vi "ReadDough.vi"(8 "error in (no error)":errorcluster, 11 "object in":refnum<class "Pizza.lvclass">) -> (0 "error out":errorcluster, 2 "dough":string, 3 "object out":refnum<class "Pizza.lvclass">)   [LabVIEW 2021, in "Pizza.lvclass"]
uses:
  Pizza.lvclass
  Pizza.lvclass/Pizza.ctl
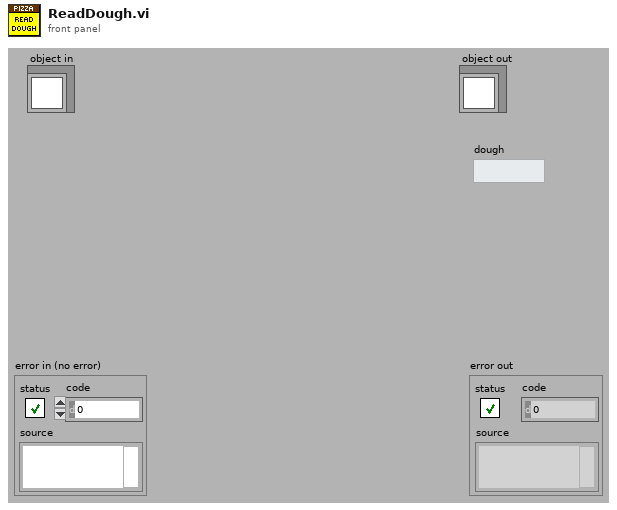
[diagram p1: front panel]
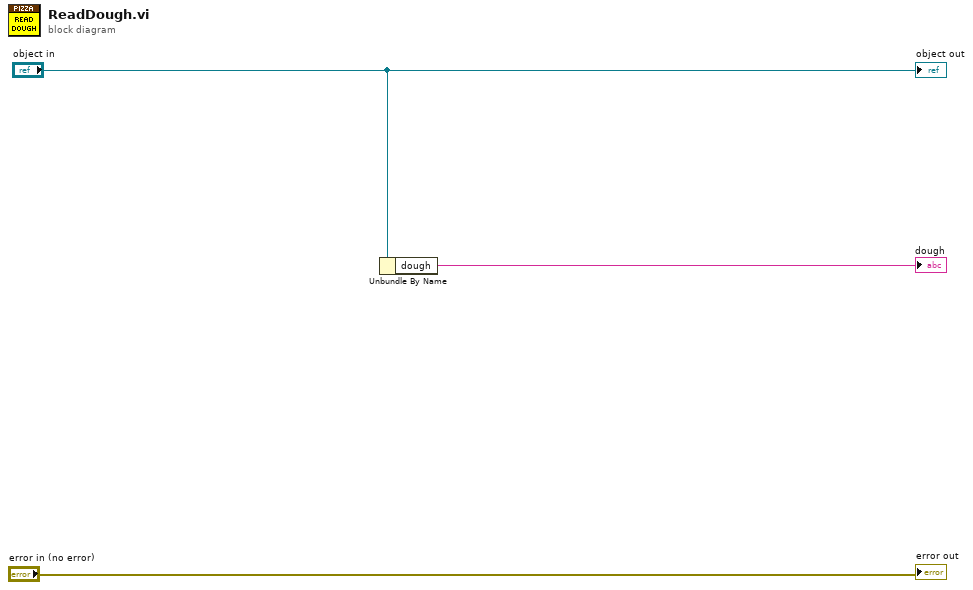
[diagram p0: block diagram]
diagram:
  n1 = Unbundle By Name("object in") -> ("dough"=→"dough":string)
  "error out" <- "error in (no error)"
  "object out" <- "object in"
